vi "onCheckConnection.vi"(8 "error in (no error)":errorcluster, 11 "Connection.LocalQueue":refnum<class "Connection.LocalQueue.lvclass">) -> (0 "error out":errorcluster, 1 "Outbound connection OK":bool, 2 "Inbound connection OK":bool, 3 "Connection.LocalQueue":refnum<class "Connection.LocalQueue.lvclass">)   [LabVIEW 2013, in "Connection.Queue_GOSPL.lvlib" / "Connection.LocalQueue.lvclass"]
uses:
  Connection.LocalQueue.lvclass
  Connection.LocalQueue.lvclass/Connection.LocalQueue.ctl
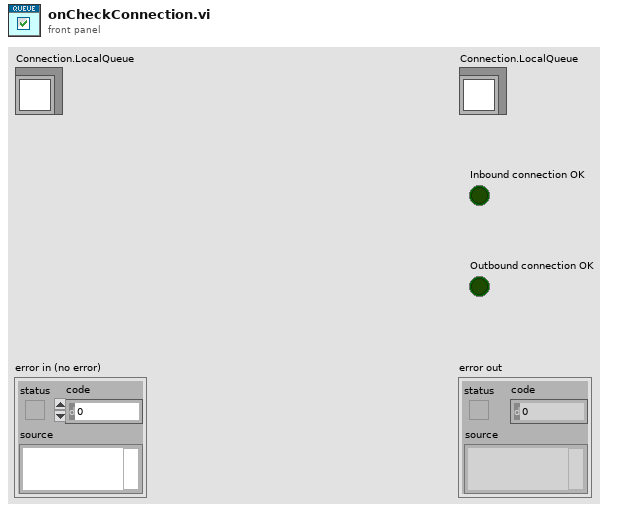
[diagram p1: front panel]
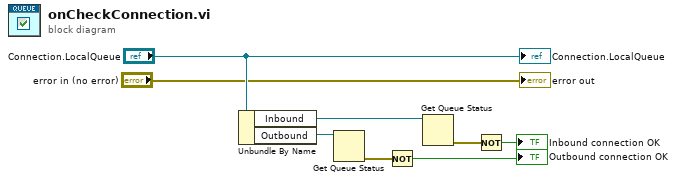
[diagram p0: block diagram]
diagram:
  n1 = Unbundle By Name("Connection.LocalQueue") -> ("Inbound"=w2:refnum<queue>, "Outbound"=w8:refnum<queue>)
  n2 = Get Queue Status(queue=w8) -> (error out=w7:errorcluster)  [unwired: 2 in, 7 out]
  n3 = Not(x=w7) -> (.not. x?=→"Outbound connection OK":bool)
  n4 = Get Queue Status(queue=w2) -> (error out=w3:errorcluster)  [unwired: 2 in, 7 out]
  n5 = Not(x=w3) -> (.not. x?=→"Inbound connection OK":bool)
  "error out" <- "error in (no error)"
  "Connection.LocalQueue" <- "Connection.LocalQueue"
